vi "Select OPC tag.vi"(9 "period":T1, 10 "access level":T2=enum."read-only", 11 "OPC Params":T3[](array[typedef]) {"data type" items=["Boolean"=1, "SByte"=2, "Byte"=3, "Int16"=4, "UInt16"=5, "Int32"=6, "UInt32"=7, "Int64"=8, "UInt64"=9, "Float"=10, "Double"=11, "String"=12, "DateTime"=13, "ByteString"=15, "Array of Boolean"=101, "Array of SByte"=102, "Array of Byte"=103, "Array of Int16"=104, "Array of UInt16"=105, "Array of Int32"=106, "Array of UInt32"=107, "Array of Int64"=108, "Array of UInt64"=109, "Array of Float"=110, "Array of Double"=111, "Array of String"=112, "Array of DateTime"=113, "Array of ByteString"=115, "Matrix of Boolean"=201, "Matrix of SByte"=202, "Matrix of Byte"=203, "Matrix of Int16"=204, "Matrix of UInt16"=205, "Matrix of Int32"=206, "Matrix of UInt32"=207, "Matrix of Int64"=208, "Matrix of UInt64"=209, "Matrix of Float"=210, "Matrix of Double"=211, "Matrix of String "=212, "Matrix of DateTime"=213, "Matrix of ByteString"=215]}) -> (3 "tags":string[](array[string]))   [LabVIEW 2019, in "OPC addons.lvlib"]
uses:
  OPC addons.lvlib
  OPC tag.ctl
  <vilib>/OPCUA/controls/Data Type.ctl
  Access level.ctl
  Period.ctl
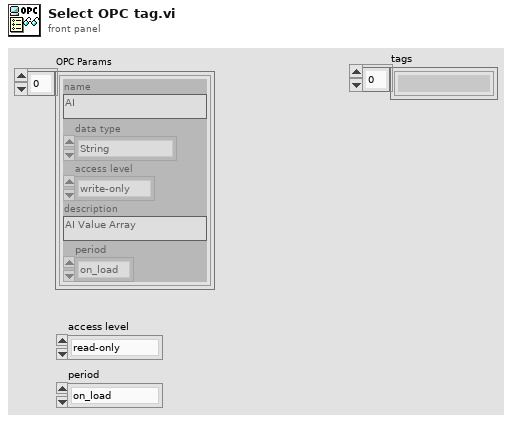
[diagram p1: front panel]
types:
  T1 = typedef "OPC addons.lvlib/Period.ctl" = enum16{"on_load", "100 ms", "500 ms", "1 s"}
  T2 = typedef "OPC addons.lvlib/Access level.ctl" = enum16{"none", "read-only", "write-only", "read/write"}
  T3 = typedef "OPC addons.lvlib/OPC tag.ctl" = cluster{"name":string, "data type":T4, "access level":T2, "description":string, "period":T1}
  T4 = typedef "Data Type.ctl" = u16
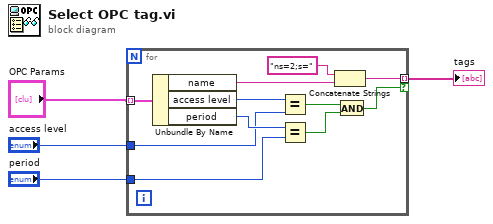
[diagram p0: block diagram]
diagram:
  n1 = for {
    tunnel: "OPC Params" -> [w14] mode=indexing
    tunnel: [w7] -> w1 mode=indexing if=w10
    tunnel: "access level" -> [w6]
    tunnel: "period" -> [w5]
    n2 = Unbundle By Name(w14) -> ("name"=w13:string, "access level"=w8:T2, "period"=w9:T1)
    n3 = Equal?(x=w8, y=w6) -> (x = y?=w12:bool)
    n4 = Equal?(x=w9, y=w5) -> (x = y?=w11:bool)
    n5 = Concatenate Strings("ns=2;s=" ("string"), w13) -> (w7:string)
    n6 = And(x=w12, y=w11) -> (x .and. y?=w10:bool)
  }
  "tags" <- w1
